vi "BoundsToJson.vi"(8 "error in (no error)":errorcluster, 10 "Owner Bounds":T1, 11 "GObj in":refnum<vi>) -> (0 "error out":errorcluster, 1 "JSON":string, 2 "Relative Bounds":cluster{"x":i32, "y":i32, "w":i32, "h":i32}, 3 "GObj out":refnum<vi>)   [LabVIEW 2017]
doc: "Converts absolute position to relative position"
uses:
  <vilib>/Utility/miscctls.llb/LVRectTypeDef.ctl
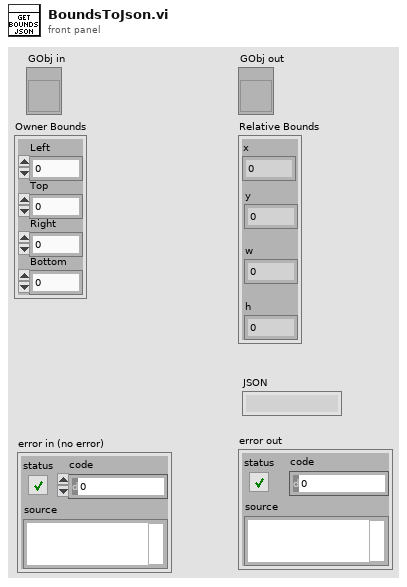
[diagram p1: front panel]
types:
  T1 = typedef "LVRectTypeDef.ctl" = cluster{"Left":i16, "Top":i16, "Right":i16, "Bottom":i16}
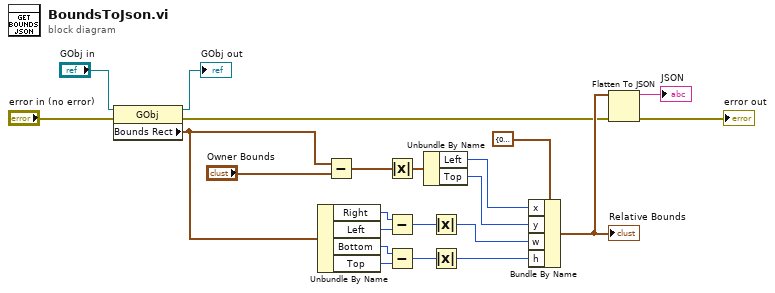
[diagram p0: block diagram]
diagram:
  n1 = property class="GObj"(reference="GObj in", error in="error in (no error)") -> (reference out=→"GObj out":refnum<vi>, error out=w4:errorcluster, "Bounds Rect"=w13:T1)
  n2 = Unbundle By Name(w13) -> ("Right"=w12:i16, "Left"=w11:i16, "Bottom"=w10:i16, "Top"=w9:i16)
  n3 = Subtract(x=w13, y="Owner Bounds") -> (x-y=w19:T1)
  n4 = Absolute Value(x=w19) -> (abs(x)=w21:T1)
  n5 = Subtract(x=w12, y=w11) -> (x-y=w8:i16)
  n6 = Subtract(x=w10, y=w9) -> (x-y=w7:i16)
  n7 = Unbundle By Name(w21) -> ("Left"=w15:i16, "Top"=w14:i16)
  n8 = Absolute Value(x=w8) -> (abs(x)=w2:i16)
  n9 = Absolute Value(x=w7) -> (abs(x)=w1:i16)
  n10 = Bundle By Name(cluster=cluster{"x":i32, "y":i32, "w":i32, "h":i32} {"x"=0, "y"=0, "w"=0, "h"=0}, "x"=w15, "y"=w14, "w"=w2, "h"=w1) -> (w6:cluster{"x":i32, "y":i32, "w":i32, "h":i32})
  "Relative Bounds" <- w6
  n11 = Flatten To JSON(anything=w6, error in (no error)=w4) -> (JSON string=→"JSON":string, 11:→"error out":errorcluster)  [unwired: 1 in]
